vi "from AtTracker format to Wilcocks format.vi"() -> ()   [LabVIEW 2010]
uses:
  <vilib>/Utility/file.llb/Write To Spreadsheet File (string).vi
  <vilib>/Utility/file.llb/Read From Spreadsheet File (string).vi
panel:
  in  "stop":bool
  out "# elements in queue":i32
  out "Files completed":i32
  out "Files to process":i32
  in  "Location to write resulting csv files into":path=path "O:/CGR2011/Processing/TESTING"
  in  "target directory to get files from":path=path "O:/CGR2011/Processing/TESTING"
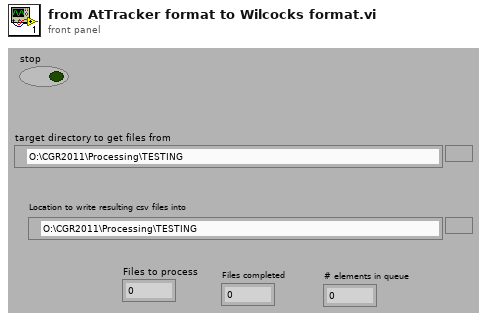
[diagram p1: front panel]
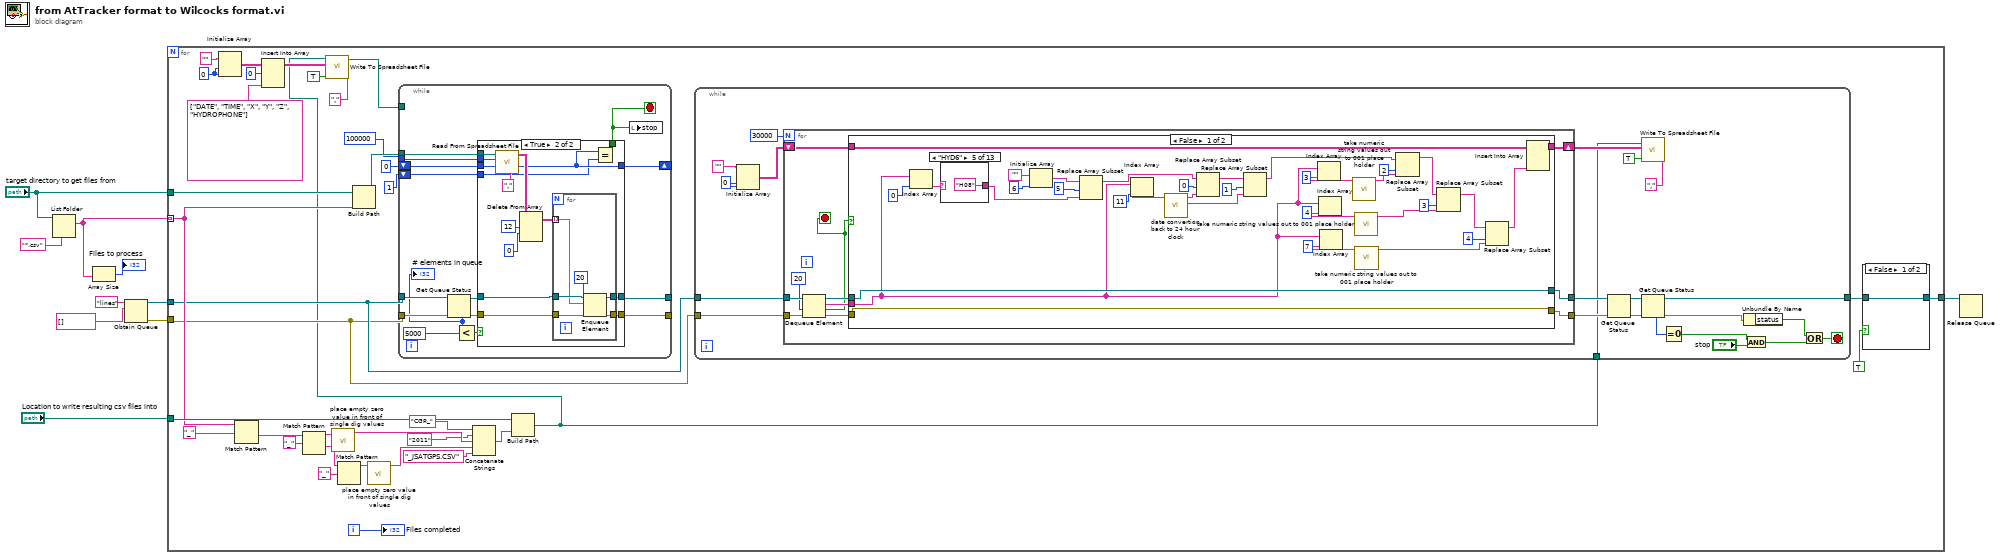
[diagram p0: block diagram]
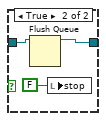
[diagram p2: hidden frame]
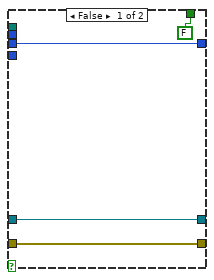
[diagram p3: hidden frame]
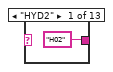
[diagram p4: hidden frame]
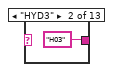
[diagram p5: hidden frame]
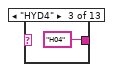
[diagram p6: hidden frame]
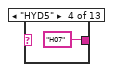
[diagram p7: hidden frame]
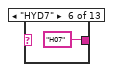
[diagram p8: hidden frame]
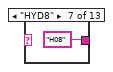
[diagram p9: hidden frame]
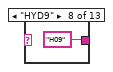
[diagram p10: hidden frame]
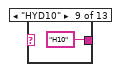
[diagram p11: hidden frame]
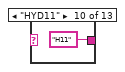
[diagram p12: hidden frame]
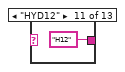
[diagram p13: hidden frame]
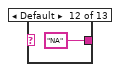
[diagram p14: hidden frame]
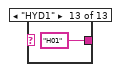
[diagram p15: hidden frame]
diagram:
  n1 = List Folder(path="target directory to get files from", pattern="*.csv") -> (filenames=w7:string[])  [unwired: 2 in, 3 out]
  n2 = Array Size(array=w7) -> (size(s)=→"Files to process":i32)
  n3 = Obtain Queue(name (unnamed)="lines", element data type=string[] [] ("all rows")) -> (queue out=w3:refnum<queue>, error out=w2:errorcluster)  [unwired: 3 in, 1 out]
  n4 = for {
    tunnel: w7 -> [w43] mode=indexing
    tunnel: "target directory to get files from" -> [w46]
    tunnel: "Location to write resulting csv files into" -> [w44]
    tunnel: w3 -> [w25]
    tunnel: w2 -> [w24]
    tunnel: [w12] -> w1
    i -> [w29]
    w16 = 0 ("dimension size")
    n5 = Initialize Array("" ("String"), w16, w16) -> (w18:string[][])
    n6 = Match Pattern(string=w43, regular expression="_") -> (after substring=w39:string)  [unwired: 1 in, 3 out]
    n7 = Insert Into Array(array=w18, index (row)=0, new element=string[] ["DATE", "TIME", "X", "Y", "Z", "HYDROPHONE"]) -> (w21:string[][])  [unwired: 1 in]
    n8 = Match Pattern(string=w39, regular expression="_") -> (before substring=w37:string, after substring=w38:string)  [unwired: 1 in, 2 out]
    n9 = call "place empty zero value in front of single dig values.vi"("input string value of numeric"=w37) -> ("formated resulting string"=w36:string)  [unwired: 10 in]
    n10 = Match Pattern(string=w38, regular expression="_") -> (before substring=w35:string)  [unwired: 1 in, 3 out]
    n11 = Build Path(base path=w46, name or relative path=w43) -> (appended path=w45:path)
    n12 = call "place empty zero value in front of single dig values.vi"("input string value of numeric"=w35) -> ("formated resulting string"=w34:string)  [unwired: 10 in]
    n13 = Concatenate Strings("CGR_" ("string"), "2011" ("string"), w36, w34, "_JSATGPS.CSV" ("string")) -> (w31:string)
    n14 = Build Path(base path=w44, name or relative path=w31) -> (appended path=w15:path)
    n15 = call-poly <vilib>:"Write To Spreadsheet File.vi"("delimiter (\\t)"="," ("delimiter (\\t)"), "append to file? (new file:F)"=TRUE, "2D data"=w21, "file path (dialog if empty)"=w15) -> ("new file path (Not A Path if cancelled)"=w14:path)  [unwired: 4 in]
    n16 = while {
      tunnel: w45 -> [w65]
      tunnel: w25 -> [w61]
      tunnel: w24 -> [w62]
      tunnel: [w64] -> _
      tunnel: [w63] -> _
      tunnel: 100000 ("number of rows (all:-1)") -> [w57]
      shift-right: [w58] -> _
      shift-left: 0 ("start of read offset (chars.:0)") -> [w56]
      shift-left: 1 ("start of read offset (chars.:0)") -> [w52]
      tunnel: w14 -> [_]
      stop <- w51 stop-if-true
      n17 = Get Queue Status(queue=w61, error in (no error)=w62) -> (queue out=w60:refnum<queue>, error out=w59:errorcluster, # elements in queue=w53:i32)  [unwired: 1 in, 5 out]
      "# elements in queue" <- w53
      n18 = Less?(x=w53, y=5000) -> (x < y?=w55:bool)
      n19 = case shown="True" w55 {
        tunnel: w65 -> [_ w84]
        tunnel: [w68 w78] -> w64
        tunnel: [w67 w77] -> w63
        tunnel: w60 -> [w68 w76]
        tunnel: w59 -> [w67 w75]
        tunnel: w57 -> [_ w74]
        tunnel: [w69 w71] -> w58
        tunnel: w56 -> [w69 w73]
        tunnel: [FALSE w72] -> w51
        tunnel: w52 -> [_ w70]
        frame False {
        }
        frame True {
          n20 = call-poly <vilib>:"Read From Spreadsheet File.vi"("delimiter (\\t)"="," ("delimiter (\\t)"), "start of read offset (chars.:0)"=w73, "number of rows (all:-1)"=w74, "file path (dialog if empty)"=w84) -> ("mark after read (chars.)"=w71:i32, "all rows"=w82:string[][])  [unwired: 3 in, 3 out]
          n21 = Delete From Array(array=w82, length=12, index (row)=0) -> (array with subset deleted=w79:string[][])  [unwired: 1 in, 1 out]
          n22 = for {
            tunnel: w79 -> [w89] mode=indexing
            tunnel: w76 -> [w90]
            tunnel: w75 -> [w88]
            tunnel: [w87] -> w78
            tunnel: [w86] -> w77
            n23 = Enqueue Element(queue=w90, element=w89, timeout in ms (-1)=20, error in (no error)=w88) -> (queue out=w87:refnum<queue>, error out=w86:errorcluster)  [unwired: 1 out]
          }
          n24 = Equal?(x=w71, y=w70) -> (x = y?=w72:bool)
        }
      }
      n25 = local write "stop"(w51) -> ()
    }
    n26 = while {
      tunnel: w25 -> [w112]
      tunnel: w24 -> [w111]
      tunnel: w15 -> [w106]
      tunnel: [w92] -> w13
      stop <- w100 stop-if-true
      w104 = 0 ("dimension size")
      n27 = Initialize Array("" ("String"), w104, w104) -> (w102:string[][])
      n28 = for {
        N: 30000 -> [_]
        tunnel: w112 -> [w119]
        tunnel: w111 -> [w118]
        tunnel: [w123] -> w110
        tunnel: [w122] -> w109
        shift-right: [w121] -> w107
        shift-left: w102 -> [w120]
        stop <- w113 stop-if-true
        n29 = Dequeue Element(queue=w119, timeout in ms (-1)=20, error in (no error)=w118) -> (queue out=w117:refnum<queue>, element=w115:string[], timed out?=w113:bool, error out=w116:errorcluster)
        n30 = case shown="False" w113 {
          tunnel: [w126 w174] -> w123
          tunnel: [w125 w173] -> w122
          tunnel: [w129 w175] -> w121
          tunnel: w120 -> [w128 w175]
          tunnel: w117 -> [w126 w174]
          tunnel: w116 -> [w125 w173]
          tunnel: w115 -> [w124 _]
          frame False {
            n31 = Index Array(array=w124, index=0) -> (element=w157:string)
            n32 = case shown="\"HYD6\"" w157 {
              tunnel: ["H02" "H03" "H04" "H07" "H08" "H07" "H08" "H09" "H10" "H11" "H12" "NA" "H01"] -> w155
              frame "HYD2" {
              }
              frame "HYD3" {
              }
              frame "HYD4" {
              }
              frame "HYD5" {
              }
              frame "HYD6" {
              }
              frame "HYD7" {
              }
              frame "HYD8" {
              }
              frame "HYD9" {
              }
              frame "HYD10" {
              }
              frame "HYD11" {
              }
              frame "HYD12" {
              }
              frame Default {
              }
              frame "HYD1" {
              }
            }
            n33 = Initialize Array("", 6 ("dimension size")) -> (w154:string[])
            n34 = Replace Array Subset(array=w154, new element=w155, index=5 ("disabled index (col)")) -> (w159:string[])
            n35 = Index Array(array=w124, index=11 ("index (row)")) -> (element=w153:string)
            n36 = call "date convertion back to 24 hour clock.vi"("DateTime as string"=w153) -> ("Time"=w150:string, "Date"=w151:string)  [unwired: 9 in]
            n37 = Replace Array Subset(array=w159, new element=w151, index=0 ("disabled index (col)")) -> (w152:string[])
            n38 = Replace Array Subset(array=w152, new element=w150, index=1 ("disabled index (col)")) -> (w158:string[])
            n39 = Index Array(array=w124, index=3 ("index (row)")) -> (element=w147:string)
            n40 = Index Array(array=w124, index=4 ("index (row)")) -> (element=w145:string)
            n41 = Index Array(array=w124, index=7 ("index (row)")) -> (element=w144:string)
            n42 = call "take numeric string values out to 001 place holder.vi"("String number out to .001"=w147) -> ("formated result"=w146:string)  [unwired: 10 in]
            n43 = call "take numeric string values out to 001 place holder.vi"("String number out to .001"=w145) -> ("formated result"=w143:string)  [unwired: 10 in]
            n44 = call "take numeric string values out to 001 place holder.vi"("String number out to .001"=w144) -> ("formated result"=w142:string)  [unwired: 10 in]
            n45 = Replace Array Subset(array=w158, new element=w146, index=2 ("disabled index (col)")) -> (w149:string[])
            n46 = Replace Array Subset(array=w149, new element=w143, index=3 ("disabled index (col)")) -> (w148:string[])
            n47 = Replace Array Subset(array=w148, new element=w142, index=4 ("disabled index (col)")) -> (w127:string[])
            n48 = Insert Into Array(array=w128, new element=w127) -> (w129:string[][])  [unwired: 2 in]
          }
          frame True {
          }
        }
      }
      n49 = Get Queue Status(queue=w110, error in (no error)=w109) -> (queue out=w95:refnum<queue>, error out=w96:errorcluster)  [unwired: 1 in, 6 out]
      n50 = call-poly <vilib>:"Write To Spreadsheet File.vi"("delimiter (\\t)"="," ("delimiter (\\t)"), "append to file? (new file:F)"=TRUE, "2D data"=w107, "file path (dialog if empty)"=w106) -> ()  [unwired: 4 in, 1 out]
      n51 = Get Queue Status(queue=w95, error in (no error)=w96) -> (queue out=w92:refnum<queue>, error out=w91:errorcluster, # elements in queue=w94:i32)  [unwired: 1 in, 5 out]
      n52 = Equal To 0?(x=w94) -> (x = 0?=w93:bool)
      n53 = Unbundle By Name(w91) -> ("status"=w99:bool)
      n54 = And(x=w93, y="stop") -> (x .and. y?=w97:bool)
      n55 = Or(x=w99, y=w97) -> (x .or. y?=w100:bool)
    }
    n56 = case shown="False" TRUE {
      tunnel: w13 -> [w47 w50]
      tunnel: [w47 w49] -> w12
      frame False {
      }
      frame True {
        n57 = Flush Queue(queue=w50) -> (queue out=w49:refnum<queue>)  [unwired: 1 in, 2 out]
        n58 = local write "stop"(FALSE ("stop")) -> ()
      }
    }
    "Files completed" <- w29
  }
  n59 = Release Queue(queue=w1) -> ()  [unwired: 2 in, 3 out]
